vi "Wrapper.vi"(0 "Spk Cycle MSG in":refnum<class "Spk Cycle MSG.lvclass">, 1 "Instrument Lib:Instr":refnum<class "Instr Actor.lvclass">, 2 "Actor in":refnum<class "Actor.lvclass">, 5 "error in (no error)":errorcluster) -> (14 "Instr Actor out":refnum<class "Instr Actor.lvclass">, 19 "error out":errorcluster)   [LabVIEW 2014, in "ePAS Library.lvlib" / "Spk Cycle MSG.lvclass"]
uses:
  Speaker Cycle MSG/Spk Cycle MSG.lvclass
  Instr Actor.lvclass
  <vilib>/ActorFramework/Actor/Actor.lvclass
  PAS/Commands/Change Speaker Switch State/Change Speaker Switch State.lvclass
  Speaker Cycle MSG/Spk Cycle MSG.lvclass/Spk Cycle MSG.ctl
  PAS/Commands/Change Speaker Switch State/Change Speaker Switch State.lvclass/Change Speaker Switch State.ctl
  PAS/Commands/Change Speaker Switch State/Write Cycle.vi
  PAS/Commands/Change Speaker Switch State/Write Period.vi
  PAS/Commands/Change Speaker Switch State/Write Length.vi
  Accessors/Read CMD.vi
  reusable/Command/Command.lvclass
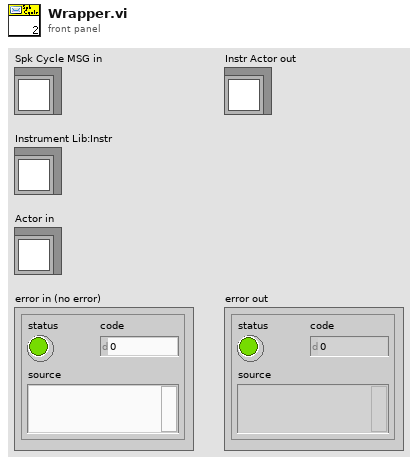
[diagram p1: front panel]
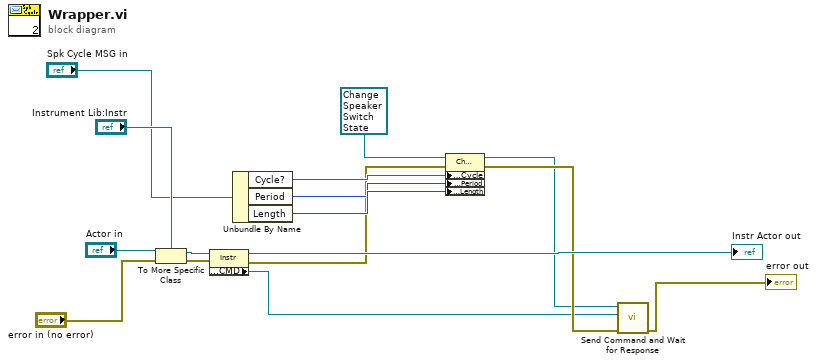
[diagram p0: block diagram]
diagram:
  n1 = To More Specific Class(target class="Instrument Lib:Instr", reference="Actor in", error in="error in (no error)") -> (specific class reference=w5:refnum<class "Instr Actor.lvclass">, error out=w16:errorcluster)
  n2 = property class="Instr"(reference=w5, error in=w16) -> (reference out=→"Instr Actor out":refnum<class "Instr Actor.lvclass">, error out=w7:errorcluster, "Accessors:CMD"=w9:refnum<queue>)
  n3 = Unbundle By Name("Spk Cycle MSG in") -> ("Cycle?"=w13:bool, "Period"=w14:i16, "Length"=w15:i16)
  n4 = property class="Change Speaker Switch"(reference=refnum<class "Change Speaker Switch State.lvclass"> refnum ("Change Speaker Switch"), error in=w7, "Accessors:Cycle"=w13, "Accessors:Period"=w14, "Accessors:Length"=w15) -> (reference out=w8:refnum<class "Change Speaker Switch State.lvclass">, error out=w10:errorcluster)
  n5 = call "Send Command and Wait for Response.vi"("error in"=w10, "cmd queue"=w9, "CMD in"=w8) -> ("error out"=→"error out":errorcluster)  [unwired: 6 in, 2 out]
